vi "AMB_TCP_Init_Globals.vi"(2 "CAN Port In":string="CAN0", 3 "ABM In":i16) -> (0 "BUS #":i32)   [LabVIEW 2017]
uses:
  AMB_Global.gbl.vi
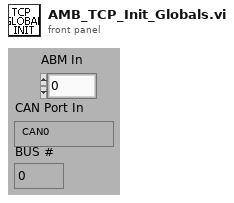
[diagram p1: front panel]
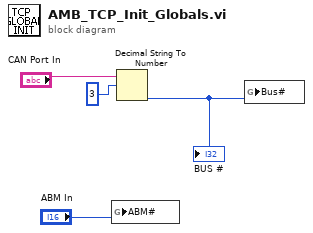
[diagram p0: block diagram]
diagram:
  n1 = global write "AMB_Global.gbl.vi" "ABM#"("ABM In") -> ()
  n2 = Decimal String To Number(string="CAN Port In", offset=3) -> (number=w1:i32)  [unwired: 1 in, 1 out]
  "BUS #" <- w1
  n3 = global write "AMB_Global.gbl.vi" "Bus#"(w1) -> ()
